vi "Send Register Event.vi"(4 "Get Last Broadcast Event (F)":bool, 5 "Event":refnum<class "Event.lvclass">, 6 "Event Handler":refnum<class "Abstract Event Message for View.lvclass">, 7 "Priority":T1=enum."Normal" caption="Message Priority (Normal)", 8 "error in (no error)":errorcluster, 11 "Message Enqueuer in":refnum<class "Message Enqueuer.lvclass">) -> (0 "error out":errorcluster, 3 "Message Enqueuer out":refnum<class "Message Enqueuer.lvclass">)   [LabVIEW 2023, in "MVC Actors.lvlib" / "Register Event Msg.lvclass"]
doc: "Sends the <b>MVC Actors.lvlib:Register Event Msg.lvclass</b> message.\n\nThis message will call <b>Register Event.vi</b> on the <b>MVC Actors.lvlib:View.lvclass</b> actor.\n\n<b>Register Event.vi Description</b>\nRegisters an event to the Controller by specifying the concrete event and the corresponding Event Handler. If \"Get Last Broadcast Event (F)\" is TRUE the View will receive the last broadcast Event."
uses:
  Register Event Msg.lvclass
  Register Event Msg.lvclass/Register Event Msg.ctl
  <vilib>/ActorFramework/Message Enqueuer/Message Enqueuer.lvclass
  C:/Program Files/National Instruments/LabVIEW 2023/vi.lib/ActorFramework/Message/Message.lvclass
  C:/Projects/Shared Libraries/Event Actors/View Messages/Register Event Msg/Register Event Msg.lvclass
  <vilib>/ActorFramework/Message Enqueuer/Message Priority.ctl
  Event/Event.lvclass
  Event Handlers/Abstract Event Message for View/Abstract Event Message for View.lvclass
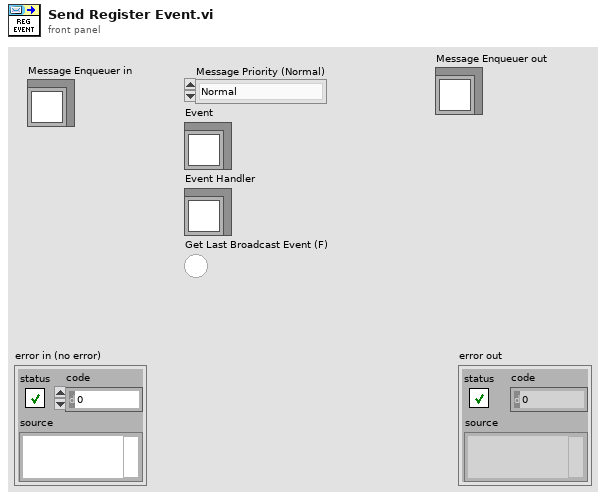
[diagram p1: front panel]
types:
  T1 = typedef "Actor Framework.lvlib/Message Enqueuer.lvclass/Message Priority.ctl" = enum16{"Low", "Normal", "High"}
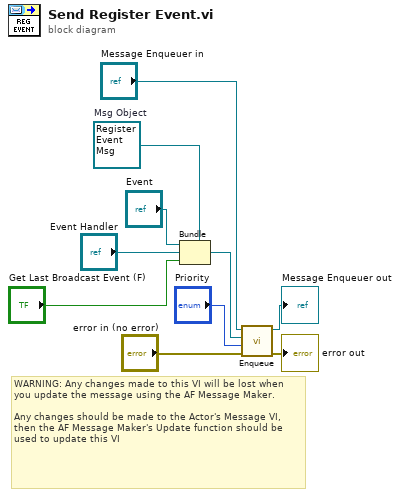
[diagram p0: block diagram]
diagram:
  w7 = refnum<class "Register Event Msg.lvclass"> refnum  # Msg Object
  # "WARNING: Any changes made to this VI will be lost when you update the message using the AF Message Maker.\n\nAny changes should be made to the Actor's Message VI, then the AF Message Maker's Update function should be used to update this VI"
  n1 = Bundle(cluster=w7, "Event", "Event Handler", "Get Last Broadcast Event (F)") -> (w2:refnum<class "Register Event Msg.lvclass">)
  n2 = call <vilib>:"Enqueue.vi"("error in (no error)"="error in (no error)", "Message Priority (Normal)"="Priority", "Message"=w2, "Message Enqueuer in"="Message Enqueuer in") -> ("error out"=→"error out":errorcluster, "Message Enqueuer out"=→"Message Enqueuer out":refnum<class "Message Enqueuer.lvclass">)  [unwired: 6 in]
